vi "Auto_Routine_RightTwoPieceTRAJ.vi"   [LabVIEW 2023]
uses:
  Shoulder/ShoulderGetSetpointEnum.ctl
  Trajectory/TrajectoryGlobals.vi
  <vilib>/Rock Robotics/WPI/ThirdParty/JAS_Junk/TrajLib/Trajectory_Library.lvlib
types:
  T1 = typedef "ShoulderGetSetpointEnum.ctl" = enum16{"ShoulderRest", "ShoulderShoot", "ShoulderAmp", "ArmFloorPickup", "ArmAmpDeposit", "ArmSpeakerShoot", "ArmStartPosition", "ArmRestPosition", "ArmSourceIntake", "ArmAwayShoot"}
  T2 = typedef "Trajectory_Library.lvlib/TRAJECTORY.ctl" = cluster{"TotalTImeSecs":dbl, "States":T3[]}
  T3 = typedef "Trajectory_Library.lvlib/TRAJ_STATE.ctl" = cluster{"TimeSeconds":dbl, "Velocity":dbl, "Acceleration":dbl, "POSE":T4, "Curvature":dbl}
  T4 = typedef "Trajectory_Library.lvlib/POSE2D.ctl" = cluster{"TRANSLATION":T5, "ROTATION":T6}
  T5 = typedef "Trajectory_Library.lvlib/TRANSLATION2D.ctl" = cluster{"X":dbl, "Y":dbl}
  T6 = typedef "Trajectory_Library.lvlib/ROTATION2D.ctl" = cluster{"VALUE":dbl, "COS":dbl, "SIN":dbl}
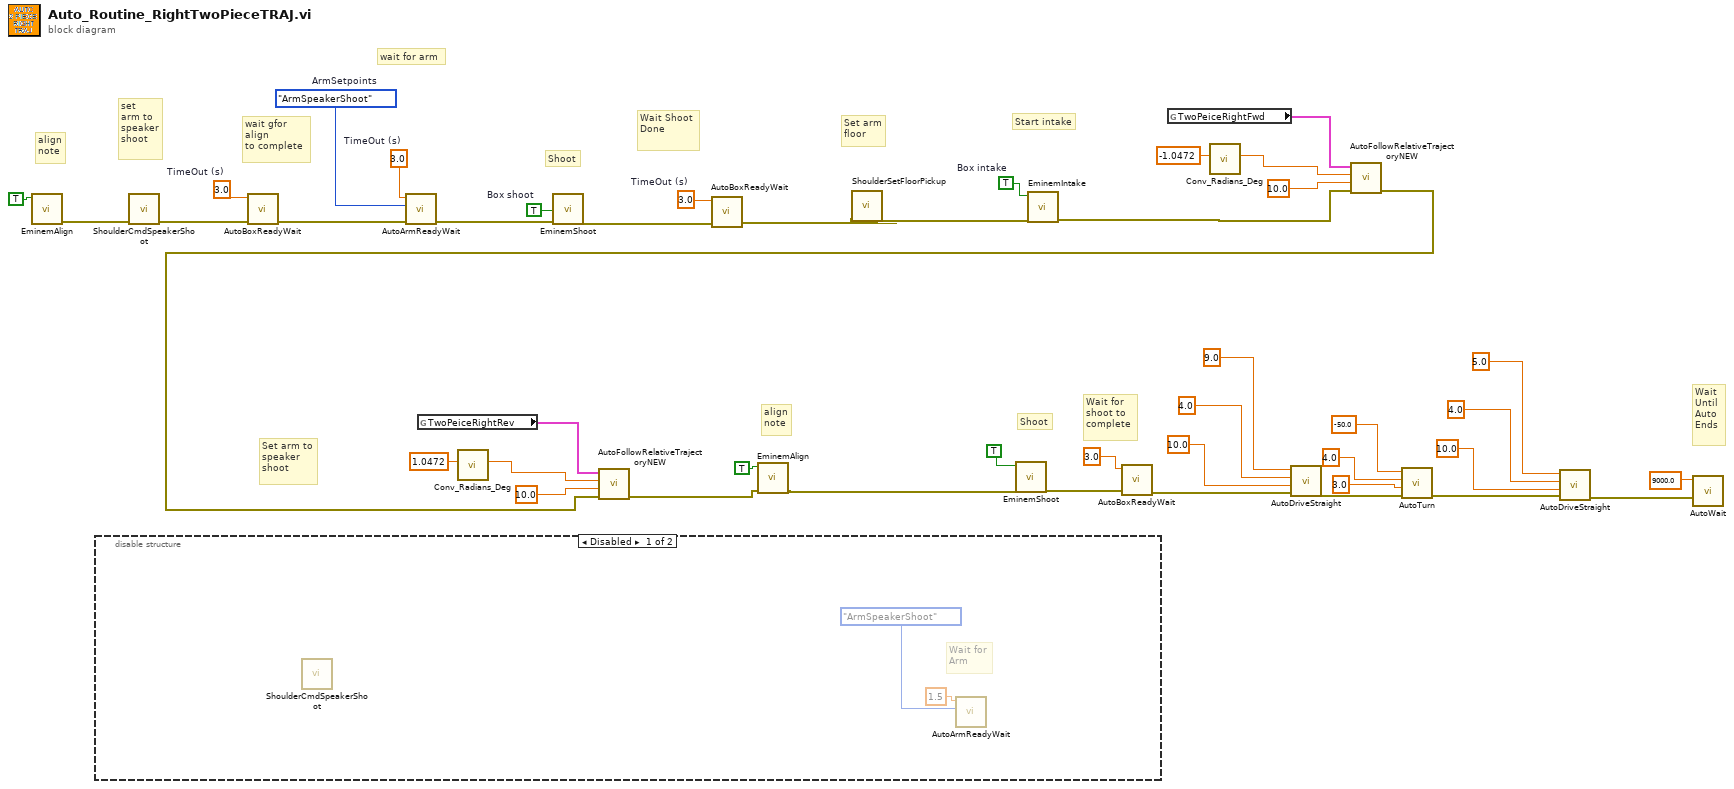
[diagram p0: block diagram]
diagram:
  w34 = 3.0  # TimeOut (s)
  w44 = TRUE  # Box intake
  w43 = TRUE  # Box shoot
  w42 = ShoulderGetSetpointEnum."ArmSpeakerShoot"  # ArmSetpoints
  w41 = 3.0  # TimeOut (s)
  w37 = 3.0  # TimeOut (s)
  # "align\nnote"
  # "Wait\nUntil\nAuto \nEnds"
  # "Wait for\nshoot to\ncomplete"
  # "Shoot"
  # "Set arm to\nspeaker \nshoot"
  # "Start intake"
  # "Set arm\nfloor"
  # "Wait Shoot\nDone"
  # "Shoot"
  # "wait gfor\nalign\nto complete"
  # "set \narm to\nspeaker\nshoot"
  # "align\nnote"
  # "wait for arm"
  n1 = call "EminemAlign.vi"("box align"=TRUE) -> ("error out"=w35:errorcluster)  [unwired: 10 in]
  n2 = disable-structure shown="Disabled" {
    frame Disabled {
      # "Wait for\nArm"
      n3 = call "ShoulderCmdSpeakerShoot.vi"() -> ()  [unwired: 11 in, 1 out]
      n4 = call "AutoArmReadyWait.vi"("ArmSetpoints"=ShoulderGetSetpointEnum."ArmSpeakerShoot", "TimeOut (s)"=1.5) -> ("error in (no error)"=w45:errorcluster)  [unwired: 8 in, 1 out]
    }
    frame Enabled {
    }
  }
  n5 = call "ShoulderCmdSpeakerShoot.vi"("error in (no error)"=w35) -> ("error out"=w33:errorcluster)  [unwired: 10 in]
  n6 = call "AutoBoxReadyWait.vi"("error in (no error)"=w33, "TimeOut (s)"=w34) -> ("error out"=w32:errorcluster)  [unwired: 9 in]
  n7 = call "AutoArmReadyWait.vi"("error in (no error)"=w32, "ArmSetpoints"=w42, "TimeOut (s)"=w41) -> ("error out"=w38:errorcluster)  [unwired: 8 in]
  n8 = global read "TrajectoryGlobals.vi" "TwoPeiceRightRev"() -> (w21:T2)
  n9 = call <vilib>:"Conv_Radians_Deg.vi"("Radians"=1.0472) -> ("Degrees"=w19:dbl)  [unwired: 10 in]
  n10 = call "EminemShoot.vi"("error in (no error)"=w38, "Box shoot"=w43) -> ("error out"=w39:errorcluster)  [unwired: 9 in]
  n11 = call "AutoBoxReadyWait.vi"("error in (no error)"=w39, "TimeOut (s)"=w37) -> ("error out"=w31:errorcluster)  [unwired: 9 in]
  n12 = call "ShoulderSetFloorPickup.vi"("error in (no error)"=w31) -> ("error out"=w40:errorcluster)  [unwired: 10 in]
  n13 = call "EminemIntake.vi"("error in (no error)"=w40, "Box intake"=w44) -> ("error out"=w30:errorcluster)  [unwired: 9 in]
  n14 = global read "TrajectoryGlobals.vi" "TwoPeiceRightFwd"() -> (w29:T2)
  n15 = call <vilib>:"Conv_Radians_Deg.vi"("Radians"=-1.0472) -> ("Degrees"=w27:dbl)  [unwired: 10 in]
  n16 = call "AutoFollowRelativeTrajectoryNEW.vi"("error in (no error)"=w30, "TimeOut (s)"=10.0, "End Orientation"=w27, "Trajectory"=w29) -> ("error out"=w2:errorcluster)  [unwired: 7 in]
  n17 = call "AutoFollowRelativeTrajectoryNEW.vi"("error in (no error)"=w2, "TimeOut (s)"=10.0, "End Orientation"=w19, "Trajectory"=w21) -> ("error out"=w12:errorcluster)  [unwired: 7 in]
  n18 = call "EminemAlign.vi"("error in (no error)"=w12, "box align"=TRUE) -> ("error out"=w1:errorcluster)  [unwired: 9 in]
  n19 = call "EminemShoot.vi"("error in (no error)"=w1, "Box shoot"=TRUE) -> ("error out"=w24:errorcluster)  [unwired: 9 in]
  n20 = call "AutoBoxReadyWait.vi"("error in (no error)"=w24, "TimeOut (s)"=3.0) -> ("error out"=w17:errorcluster)  [unwired: 9 in]
  n21 = call "AutoDriveStraight.vi"("error in (no error)"=w17, "TimeOut (s)"=10.0, "MaxSpeed (ft/s)"=4.0, "Dist (ft)"=9.0) -> ("error out"=w6:errorcluster)  [unwired: 7 in]
  n22 = call "AutoTurn.vi"("error in (no error)"=w6, "TimeOut (s)"=3.0, "MaxSpeed (ft/s)"=4.0, "degrees"=-50.0) -> ("error out"=w8:errorcluster)  [unwired: 7 in]
  n23 = call "AutoDriveStraight.vi"("error in (no error)"=w8, "TimeOut (s)"=10.0, "MaxSpeed (ft/s)"=4.0, "Dist (ft)"=5.0) -> ("error out"=w7:errorcluster)  [unwired: 7 in]
  n24 = call "AutoWait.vi"("error in (no error)"=w7, "TimeOut (s)"=9000.0) -> ()  [unwired: 9 in, 1 out]
